vi "Write Value (variant).vi"(8 "error in (no error)":errorcluster, 10 "Variant":variant, 11 "U32 D Element in":refnum<class "U32 D Element.lvclass">) -> (0 "error out":errorcluster, 3 "U32 D Element out":refnum<class "U32 D Element.lvclass">)   [LabVIEW 2018, in "D Datagrid Library.lvlib" / "U32 D Element.lvclass"]
uses:
  U32 D Element.lvclass
  U32 D Element.lvclass/U32 D Element.ctl
  Write Value.vi
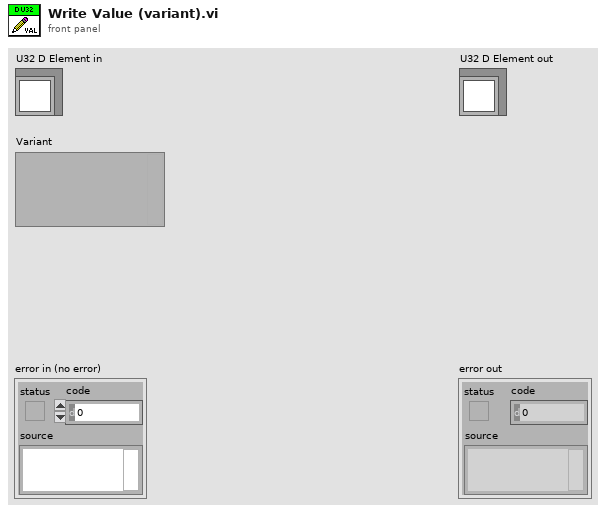
[diagram p1: front panel]
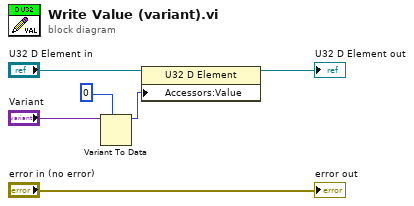
[diagram p0: block diagram]
diagram:
  n1 = Variant To Data(type=u32 0 ("Value"), Variant="Variant") -> (data=w1:u32)  [unwired: 1 in, 1 out]
  n2 = property class="U32 D Element"(reference="U32 D Element in", "Accessors:Value"=w1) -> (reference out=→"U32 D Element out":refnum<class "U32 D Element.lvclass">)  [unwired: 1 in, 1 out]
  "error out" <- "error in (no error)"
